vi "GD_All.vi"(8 "error in (no error)":errorcluster, 11 "DBlink":string="Driver={ODBC Driver 17 for SQL Server};Server=localhost\\SQLEXPRESS;Database=ZDX201;UID=labview;PWD=Dsa@54137926") -> (0 "error out":errorcluster={"status"=TRUE, "code"=-2147217843, "source"="NI_Database_API.lvlib:DB Tools Open Connec (String).vi->WD_assemble_data.vi<ERR>ADO Error: 0x80040E4D\r\nException occured in Microsoft OLE DB Provider for ODBC Drivers: [Microsoft][ODBC Driver 17 for SQL Server][SQL Server]使用者 'labview' 的登入失敗。 in NI_Database_API.lvlib:DB Tools Open Connec (String).vi->WD_assemble_data.vi"}, 3 "Workplace":T3(array[cluster]))   [LabVIEW 2019]
uses:
  <vilib>/addons/database/Auxilliary.llb/DB Tools DataTypes.ctl
  <vilib>/addons/database/Connection.llb/DB Tools Open Connec (String).vi
  <vilib>/addons/database/Connection.llb/Conn Execute.vi
  <vilib>/addons/database/Recordset.llb/Rec Fetch Recordset Data (R).vi
  <vilib>/addons/database/Recordset.llb/Rec Destroy - Connection.vi
  <vilib>/addons/database/_DB Variant To Data/Database Variant To Data.xnode
  <vilib>/addons/database/NI_Database_API.lvlib
panel:
  out "column information":T2(array[cluster])=[{"name"="assemble_Tray", "database data type"=enum."Long (I32)", "defined size"=1}, {"name"="screw_A_Tray", "database data type"=enum."Long (I32)", "defined size"=1}, {"name"="screw_B_Tray", "database data type"=enum."Long (I32)", "defined size"=1}]
  out "查詢結果":string="SELECT [id]\n      ,[name]\n      ,[barcode A]\n      ,[barcode B]\n      ,[update_time]\n  FROM [ZDX201].[dbo].[workplace_data]\n  where id>0 and id<6\n  order by id"
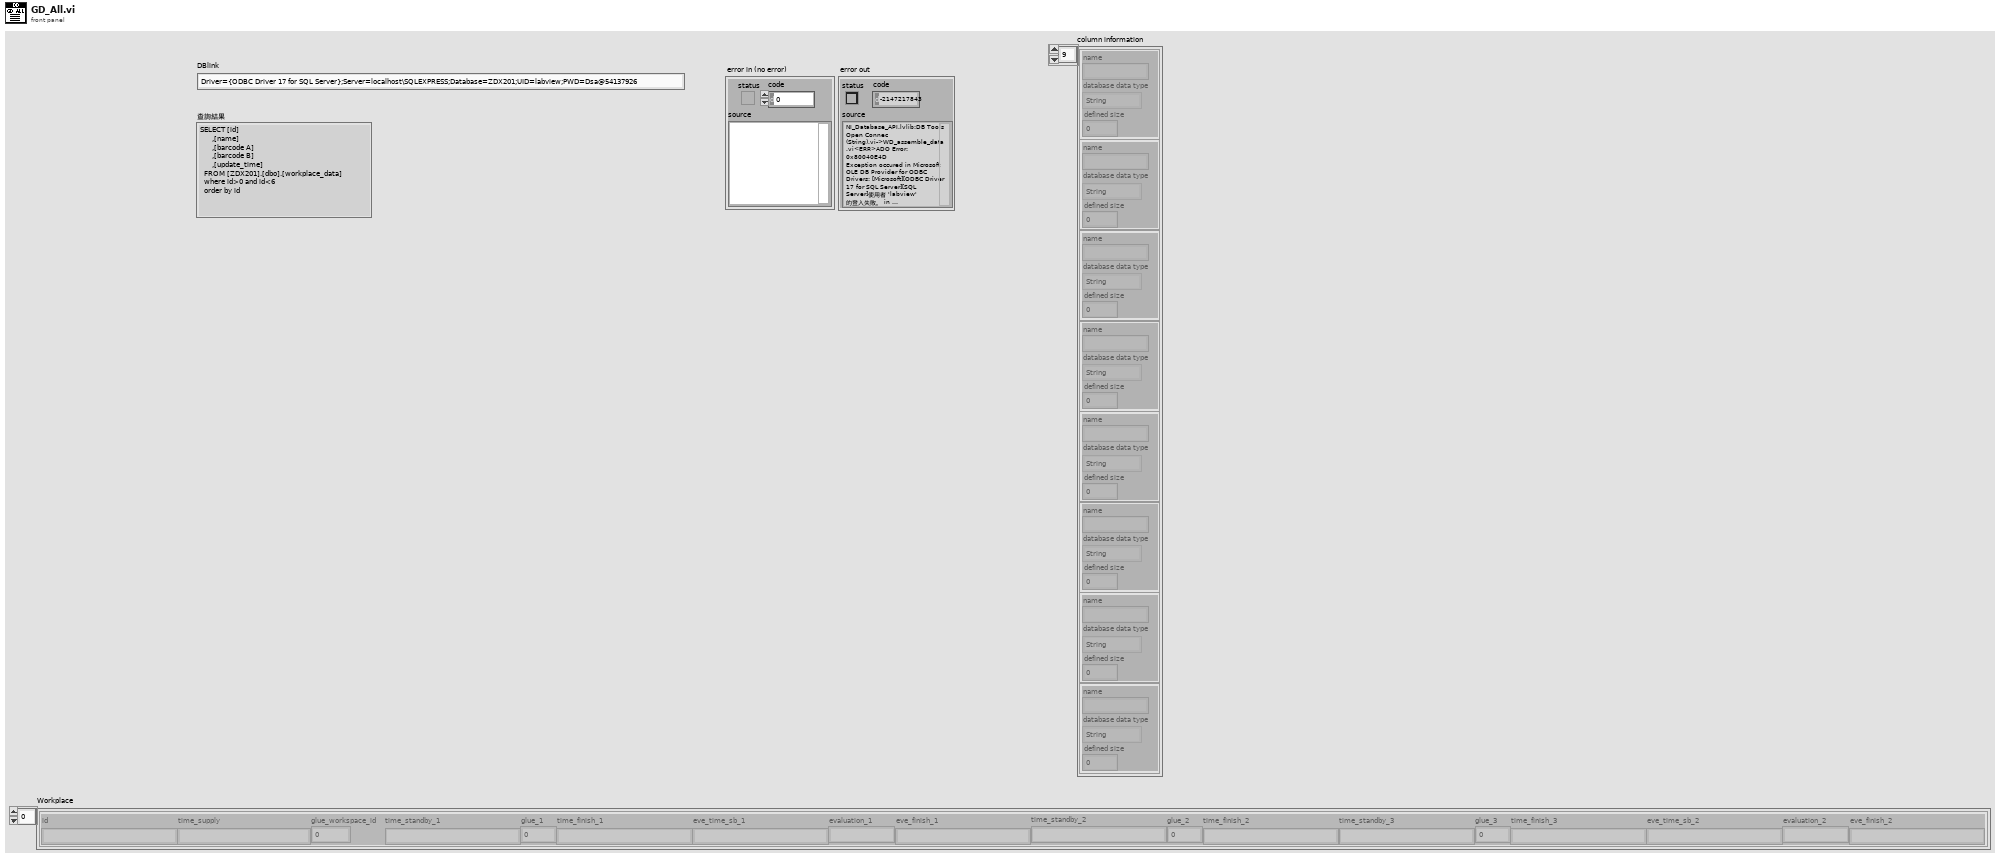
[diagram p1: front panel]
types:
  T1 = typedef "NI_Database_API.lvlib/DB Tools DataTypes.ctl" = enum16{"String", "Long (I32)", "Single (SGL)", "Double (DBL)", "Date/Time", "Binary"}
  T2 = cluster{"name":string, "database data type":T1, "defined size":i32}[]
  T3 = cluster{"id":string, "time_supply":string, "glue_workspace_id":i16, "time_standby_1":string, "glue_1":dbl, "time_finish_1":string, "eve_time_sb_1":string, "evaluation_1":string, "eve_finish_1":string, "time_standby_2":string, "glue_2":dbl, "time_finish_2":string, "time_standby_3":string, "glue_3":dbl, "time_finish_3":string, "eve_time_sb_2":string, "evaluation_2":string, "eve_finish_2":string}[]
  T4 = typedef "NI_Database_API.lvlib/Conn ObjectReference.ctl" = refnum<k1>
  T5 = typedef "NI_Database_API.lvlib/Rec ObjectReference.ctl" = refnum<k1>
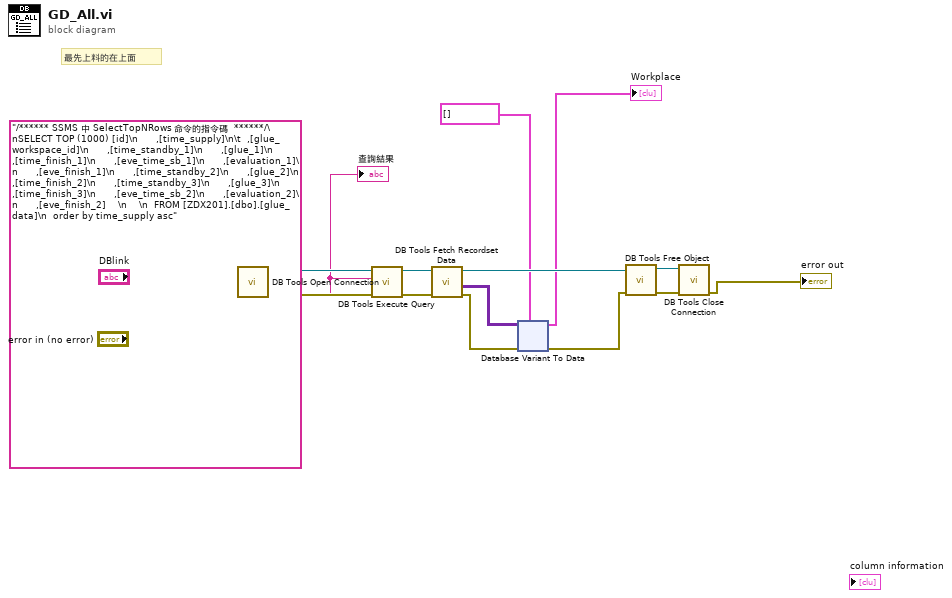
[diagram p0: block diagram]
diagram:
  w6 = "/****** SSMS 中 SelectTopNRows 命令的指令碼  ******/\nSELECT TOP (1000) [id]\n      ,[time_supply]\n\t  ,[glue_workspace_id]\n      ,[time_standby_1]\n      ,[glue_1]\n      ,[time_finish_1]\n      ,[eve_time_sb_1]\n      ,[evaluation_1]\n      ,[eve_finish_1]\n      ,[time_standby_2]\n      ,[glue_2]\n      ,[time_finish_2]\n      ,[time_standby_3]\n      ,[glue_3]\n      ,[time_finish_3]\n      ,[eve_time_sb_2]\n      ,[evaluation_2]\n      ,[eve_finish_2]    \n    \n  FROM [ZDX201].[dbo].[glue_data]\n  order by time_supply asc"
  # "最先上料的在上面"
  n1 = call-poly <vilib>:"DB Tools Open Connection.vi"("error in (no error)"="error in (no error)", "connection information"="DBlink") -> ("error out"=w16:errorcluster, "connection reference"=w15:T4)  [unwired: 6 in]
  n2 = call-poly <vilib>:"DB Tools Execute Query.vi"("error in (no error)"=w16, "SQL query"=w6, "connection reference"=w15) -> ("error out"=w13:errorcluster, "recordset reference"=w14:T5)  [unwired: 5 in]
  n3 = call-poly <vilib>:"DB Tools Fetch Recordset Data.vi"("error in (no error)"=w13, "recordset reference"=w14) -> ("error out"=w8:errorcluster, "recordset data"=w7:variant[][], "recordset reference out"=w9:T5)  [unwired: 3 in]
  n4 = xnode "Database Variant To Data"("database variant"=w7, "error in (no error)"=w8, "type"=T3 [] ("Workplace")) -> ("data"=→"Workplace":T3, "error out"=w10:errorcluster)
  n5 = call-poly <vilib>:"DB Tools Free Object.vi"("error in (no error)"=w10, "recordset reference"=w9) -> ("error out"=w11:errorcluster, "connection reference"=w12:T4)  [unwired: 8 in]
  n6 = call <vilib>:"DB Tools Close Connection.vi"("error in (no error)"=w11, "connection reference"=w12) -> ("error out"=→"error out":errorcluster)  [unwired: 5 in]
  "查詢結果" <- w6
